vi "Dual Single Gauge - Example.vi"(8 "error in (no error)":errorcluster caption="Fehler (Eingang, kein Fehler)", 11 "input refnum":refnum<visa-resource-name> caption="Eingang (Referenz)") -> (0 "error out":errorcluster, 1 "Status Sensor 2":i32(ring) items=["data OK", "underrange", "overrange", "sensor error", "sensor off", "no sensor", "ID error"], 2 "Status Sensor 1":i32(ring) items=["data OK", "underrange", "overrange", "sensor error", "sensor off", "no sensor", "ID error"], 3 "Pressure Sensor 2":dbl format="%.3e", 5 "Pressure Sensor 1":dbl format="%.3e")   [LabVIEW 2013, in "Dual Gauge.lvlib"]
uses:
  Dual Gauge.lvlib
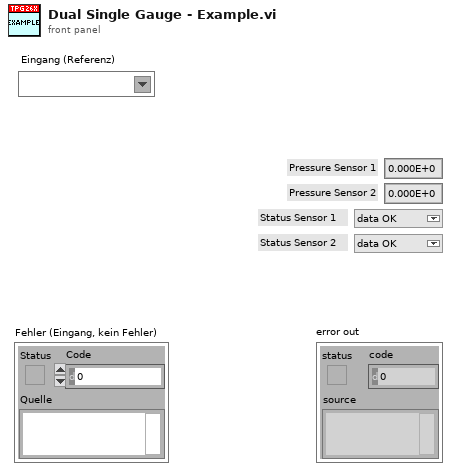
[diagram p1: front panel]
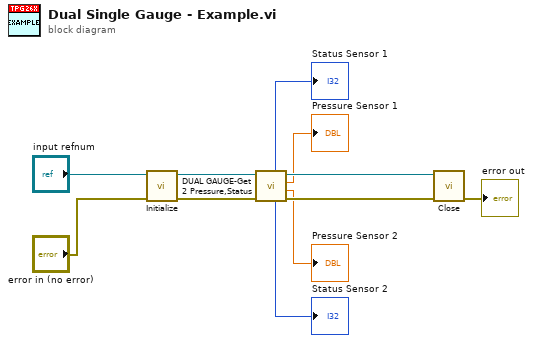
[diagram p0: block diagram]
diagram:
  n1 = call "Initialize.vi"("error in (no error)"="error in (no error)", "input refnum"="input refnum") -> ("Cluster (Ausgang)"=w6:errorcluster, "Referenz out"=w10:refnum<visa-resource-name>)  [unwired: 8 in]
  n2 = call <instrlib>:"DUAL GAUGE-Get 2 Pressure,Status.vi"("Fehler (Eingang)"=w6, "Referenz in"=w10) -> ("Cluster (Ausgang)"=w8:errorcluster, "Pressure Sensor 2"=→"Pressure Sensor 2":dbl, "Pressure Sensor 1"=→"Pressure Sensor 1":dbl, "Referenz out"=w9:refnum<visa-resource-name>, "Status Sensor 2"=→"Status Sensor 2":i32, "Status Sensor 1"=→"Status Sensor 1":i32)  [unwired: 4 in]
  n3 = call "Close.vi"("error in (no error)"=w8, "VISA resource name"=w9) -> ("error out"=→"error out":errorcluster)  [unwired: 9 in]
